vi "tm_startrecorder_40.vi"(6 "Buffering Mode":i32(ring) items=["DEFAULT", "NO BUFFERING"], 8 "error in (no error)":errorcluster, 9 "frames":i32, 10 "File":path, 11 "Handle in":u32) -> (0 "error out":errorcluster, 3 "Handle out":u32)   [LabVIEW 2023]
uses:
  tmcamcon.dll
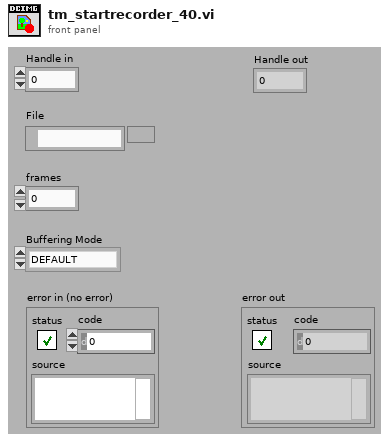
[diagram p1: front panel]
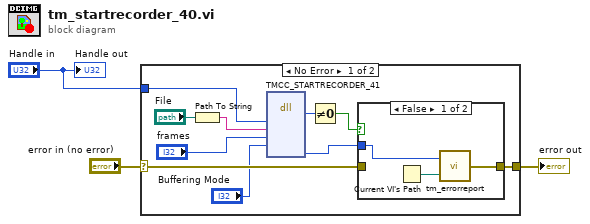
[diagram p0: block diagram]
diagram:
  n1 = case shown="No Error" "error in (no error)" {
    selector: "error in (no error)" -> [w8 w18]
    tunnel: [w5 w18] -> w2
    tunnel: "Handle in" -> [w12 _]
    frame No Error {
      n2 = Path To String(path="File") -> (string=w10:string)
      n3 = dll-call lib="tmcamcon.dll" fn="TMCC_STARTRECORDER_41"("handle"=w12, "path"=w10, "frames"="frames", "bufferingmode"="Buffering Mode") -> ("return type"=w13:u32, "Erval"=w7:i32)  [unwired: 8 in, 2 out]
      n4 = Not Equal To 0?(x=w13) -> (x != 0?=w6:bool)
      n5 = case shown="False" w6 {
        tunnel: w8 -> [_ w17]
        tunnel: [w15 w17] -> w5
        tunnel: w7 -> [w14 _]
        frame False {
          n6 = Current VI's Path() -> (path=w16:path)
          n7 = call "tm_errorreport.vi"("Source"=w16, "Error"=w14) -> ("error out"=w15:errorcluster)
        }
        frame True {
        }
      }
    }
    frame Error {
    }
  }
  "error out" <- w2
  "Handle out" <- "Handle in"
